vi "FileExistence.vi"(0 "Path":path) -> ()   [LabVIEW 2019]
uses:
  <vilib>/Utility/file.llb/Write Delimited Spreadsheet (string).vi
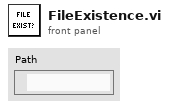
[diagram p1: front panel]
types:
  T1 = enum16{"open", "replace", "create", "open or create", "replace or create", "replace or create with confirmation"}
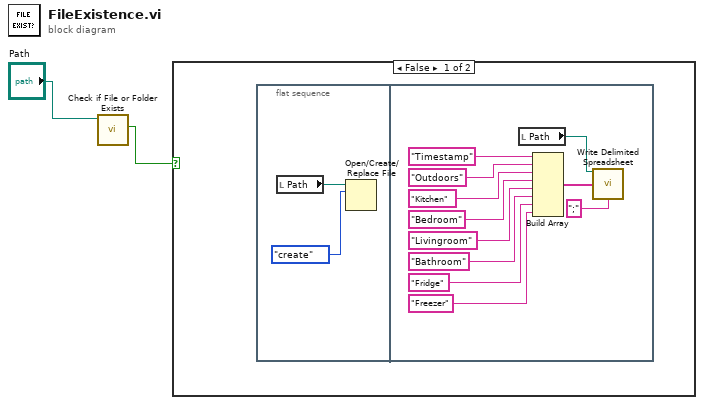
[diagram p0: block diagram]
diagram:
  n1 = call <vilib>:"Check if File or Folder Exists.vi"("path"="Path") -> ("file or folder exists?"=w2:bool)  [unwired: 8 in, 2 out]
  n2 = case shown="False" w2 {
    frame False {
      n3 = flat-sequence {
        frame #0 {
          n4 = local read "Path"() -> (w3:path)
          n5 = Open/Create/Replace File(file path (use dialog)=w3, operation (0:open)=T1."create") -> ()  [unwired: 4 in, 3 out]
        }
        frame #1 {
          n6 = local read "Path"() -> (w5:path)
          n7 = Build Array("Timestamp", "Outdoors", "Kitchen", "Bedroom", "Livingroom", "Bathroom", "Fridge", "Freezer") -> (w7:string[])
          n8 = call-poly <vilib>:"Write Delimited Spreadsheet.vi"("file path (dialog if empty)"=w5, "1D data"=w7, "delimiter (\\t)"=";" ("delimiter (\\t)")) -> ()  [unwired: 11 in, 2 out]
        }
      }
    }
    frame True {
    }
  }
